vi "VI Tree.vi"   [LabVIEW 2021, in "libad4.lvlib"]
doc: "This is the instrument driver for the <INSTRUMENT NAME>. The VI Tree displays all the user-callable VIs of the instrument driver in an organized table."
uses:
  <userlib>/libad4/libad4.lvlib
panel:
  # "SEE DIAGRAM\nFOR VI TREE."
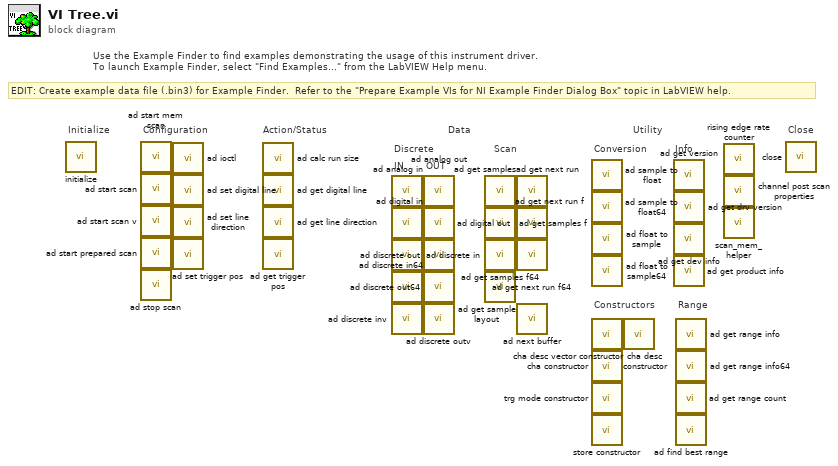
[diagram p0: block diagram]
diagram:
  # "Range"
  # "Info"
  # "Conversion"
  # "Constructors"
  # "Scan"
  # "OUT"
  # "IN"
  # "Discrete"
  # "EDIT: Create example data file (.bin3) for Example Finder.  Refer to the \"Prepare Example VIs for NI Example Finder Dialog Box\" topic in LabVIEW help."
  # "Use the Example Finder to find examples demonstrating the usage of this instrument driver.\nTo launch Example Finder, select \"Find Examples...\" from the LabVIEW Help menu."
  # "Configuration"
  # "Utility"
  # "Data"
  # "Action/Status"
  # "Close"
  # "Initialize"
  n1 = call <userlib>:"initialize.vi"() -> ()  [unwired: 10 in, 2 out]
  n2 = call <userlib>:"ad start mem scan.vi"() -> ()  [unwired: 8 in, 4 out]
  n3 = call <userlib>:"ad start scan.vi"() -> ()  [unwired: 8 in, 4 out]
  n4 = call <userlib>:"ad start scan v.vi"() -> ()  [unwired: 12 in, 4 out]
  n5 = call <userlib>:"ad start prepared scan.vi"() -> ()  [unwired: 10 in, 2 out]
  n6 = call <userlib>:"ad stop scan.vi"() -> ()  [unwired: 9 in, 3 out]
  n7 = call <userlib>:"ad ioctl.vi"() -> ()  [unwired: 9 in, 3 out]
  n8 = call <userlib>:"ad set digital line.vi"() -> ()  [unwired: 10 in, 2 out]
  n9 = call <userlib>:"ad set line direction.vi"() -> ()  [unwired: 10 in, 2 out]
  n10 = call <userlib>:"ad set trigger pos.vi"() -> ()  [unwired: 9 in, 3 out]
  n11 = call <userlib>:"ad calc run size.vi"() -> ()  [unwired: 8 in, 4 out]
  n12 = call <userlib>:"ad get digital line.vi"() -> ()  [unwired: 9 in, 3 out]
  n13 = call <userlib>:"ad get line direction.vi"() -> ()  [unwired: 9 in, 3 out]
  n14 = call <userlib>:"ad get trigger pos.vi"() -> ()  [unwired: 9 in, 3 out]
  n15 = call <userlib>:"ad analog in.vi"() -> ()  [unwired: 9 in, 3 out]
  n16 = call <userlib>:"ad digital in.vi"() -> ()  [unwired: 9 in, 3 out]
  n17 = call <userlib>:"ad discrete in.vi"() -> ()  [unwired: 9 in, 3 out]
  n18 = call <userlib>:"ad discrete in64.vi"() -> ()  [unwired: 9 in, 3 out]
  n19 = call <userlib>:"ad discrete inv.vi"() -> ()  [unwired: 13 in, 3 out]
  n20 = call <userlib>:"ad analog out.vi"() -> ()  [unwired: 10 in, 2 out]
  n21 = call <userlib>:"ad digital out.vi"() -> ()  [unwired: 10 in, 2 out]
  n22 = call <userlib>:"ad discrete out.vi"() -> ()  [unwired: 10 in, 2 out]
  n23 = call <userlib>:"ad discrete out64.vi"() -> ()  [unwired: 10 in, 2 out]
  n24 = call <userlib>:"ad discrete outv.vi"() -> ()  [unwired: 14 in, 2 out]
  n25 = call <userlib>:"ad get samples.vi"() -> ()  [unwired: 12 in, 4 out]
  n26 = call <userlib>:"ad get samples f.vi"() -> ()  [unwired: 12 in, 4 out]
  n27 = call <userlib>:"ad get samples f64.vi"() -> ()  [unwired: 12 in, 4 out]
  n28 = call <userlib>:"ad get sample layout.vi"() -> ()  [unwired: 9 in, 3 out]
  n29 = call <userlib>:"ad get next run.vi"() -> ()  [unwired: 7 in, 5 out]
  n30 = call <userlib>:"ad get next run f.vi"() -> ()  [unwired: 7 in, 5 out]
  n31 = call <userlib>:"ad get next run f64.vi"() -> ()  [unwired: 7 in, 5 out]
  n32 = call <userlib>:"ad next buffer.vi"() -> ()  [unwired: 9 in, 3 out]
  n33 = call <userlib>:"ad sample to float.vi"() -> ()  [unwired: 9 in, 3 out]
  n34 = call <userlib>:"ad sample to float64.vi"() -> ()  [unwired: 9 in, 3 out]
  n35 = call <userlib>:"ad float to sample.vi"() -> ()  [unwired: 9 in, 3 out]
  n36 = call <userlib>:"ad float to sample64.vi"() -> ()  [unwired: 9 in, 3 out]
  n37 = call <userlib>:"cha desc vector constructor.vi"() -> ()  [unwired: 11 in, 1 out]
  n38 = call <userlib>:"cha constructor.vi"() -> ()  [unwired: 11 in, 1 out]
  n39 = call <userlib>:"trg mode constructor.vi"() -> ()  [unwired: 11 in, 1 out]
  n40 = call <userlib>:"store constructor.vi"() -> ()  [unwired: 11 in, 1 out]
  n41 = call <userlib>:"cha desc constructor.vi"() -> ()  [unwired: 11 in, 1 out]
  n42 = call <userlib>:"ad get version.vi"() -> ()  [unwired: 10 in, 2 out]
  n43 = call <userlib>:"ad get drv version.vi"() -> ()  [unwired: 9 in, 3 out]
  n44 = call <userlib>:"ad get dev info.vi"() -> ()  [unwired: 9 in, 3 out]
  n45 = call <userlib>:"ad get product info.vi"() -> ()  [unwired: 9 in, 3 out]
  n46 = call <userlib>:"ad get range info.vi"() -> ()  [unwired: 9 in, 3 out]
  n47 = call <userlib>:"ad get range info64.vi"() -> ()  [unwired: 9 in, 3 out]
  n48 = call <userlib>:"ad get range count.vi"() -> ()  [unwired: 10 in, 2 out]
  n49 = call <userlib>:"ad find best range.vi"() -> ()  [unwired: 9 in, 3 out]
  n50 = call <userlib>:"rising edge rate counter.vi"() -> ()  [unwired: 11 in, 1 out]
  n51 = call <userlib>:"channel post scan properties.vi"() -> ()  [unwired: 11 in, 1 out]
  n52 = call <userlib>:"scan_mem_helper.vi"() -> ()  [unwired: 8 in, 4 out]
  n53 = call <userlib>:"close.vi"() -> ()  [unwired: 10 in, 2 out]
